vi "contatore_pulsew.vi"() -> ()   [LabVIEW 2014]
doc: "Contatore di pulse width\nFN & ADL febb 2012"
uses:
  <vilib>/DAQmx/read.llb/DAQmx Read (Counter 1D DBL 1Chan NSamp).vi
  <vilib>/Analysis/baseanly.llb/Mean (DBL).vi
  <vilib>/DAQmx/create/channels.llb/DAQmx Create Channel (CI-Pulse Width).vi
  <vilib>/DAQmx/miscellaneous.llb/DAQmx Fill In Error Info.vi
  <vilib>/Analysis/NI_AALBase.lvlib
panel:
  out "Istogramma":T1(graph)
  out "Media":dbl format="%.3e"
  in  "Azzera la figura":bool
  in  "Starting edge":i32(ring)=10280 items=["Rising"=10280, "Falling"=10171]
  in  "Numero campioni":i32=100
  out "Waveform Chart":dbl[](graph)=[857.7892626229052, 855.230805413611, 853.9527337161888, 856.0361247244633, 857.513425444567, 856.6961512925403, 855.9720097152823, 853.3515381661476, 854.4269998931967, 855.4685829162925, 858.4059401691061, 858.2401785139573, 855.2125203112975, 855.3771143853047, 855.9536929052139, 857.0540908263073, 859.4941876705559, 857.7340809915407, 855.5875212560026, 853.5245228264465, 855.8071866408499, 857.311257568451, 856.5402199167015, 856.0727661851258, 853.7704638108045, 853.4789937482665, 855.2125203112975, 858.1020926964785, 858.2493858152833, 855.8987471782089, 855.1302470257501, 856.0727661851258, 856.3018464008563, 859.2633964533904, 858.0284650943296, 856.1643835616438, 853.752241099633, 855.3771143853047, 857.5869646781368, 856.7144998929108, 856.3018464008563, 854.3631256874954, 853.4061573254252, 855.0205739325602, 857.9180473785243, 858.5164835164836, 855.9079043094964, 855.1211065267119, 855.743105919603, 856.384345294168, 859.4757198109153, 857.9548501260122, 856.3293442658046, 853.5336292249916, 854.5912917147374, 857.2010243552241, 856.9163863835986, 855.9170616367275, 854.5730339479139, 853.0239699735562, 854.4452514205153, 857.0908194859599, 857.9732526838477, 856.0269648493928, 854.8926575406877, 855.459435182908, 855.8895902428587, 858.9866105462081, 857.568578687277, 856.1368962897168, 853.4607834769993, 854.3996240641654, 856.8429621061201, 856.8888508049399, 856.2376915831835, 855.2399482579832, 853.0967411704487, 854.417874421933, 857.1275512937269, 858.5717658674795, 856.5402199167015, 854.7008547008546, 855.6058223976214, 856.3660108330301, 858.866725355893, 858.157321690999, 856.8337849561408, 853.752241099633, 854.1442008947162, 856.9990037386582, 856.9163863835986, 856.1918725986494, 855.3222426549204, 852.5512596444862, 854.5182653279215, 856.742024267218, 858.3322604180079, 856.8429621061201, 854.837847945718, 855.4045528907328]
  out "Durata":dbl[](array[numeric])=[857.7892626229052, 855.230805413611, 853.9527337161888, 856.0361247244633, 857.513425444567, 856.6961512925403, 855.9720097152823, 853.3515381661476, 854.4269998931967, 855.4685829162925, 858.4059401691061, 858.2401785139573, 855.2125203112975, 855.3771143853047, 855.9536929052139, 857.0540908263073, 859.4941876705559, 857.7340809915407, 855.5875212560026, 853.5245228264465, 855.8071866408499, 857.311257568451, 856.5402199167015, 856.0727661851258, 853.7704638108045, 853.4789937482665, 855.2125203112975, 858.1020926964785, 858.2493858152833, 855.8987471782089, 855.1302470257501, 856.0727661851258, 856.3018464008563, 859.2633964533904, 858.0284650943296, 856.1643835616438, 853.752241099633, 855.3771143853047, 857.5869646781368, 856.7144998929108, 856.3018464008563, 854.3631256874954, 853.4061573254252, 855.0205739325602, 857.9180473785243, 858.5164835164836, 855.9079043094964, 855.1211065267119, 855.743105919603, 856.384345294168, 859.4757198109153, 857.9548501260122, 856.3293442658046, 853.5336292249916, 854.5912917147374, 857.2010243552241, 856.9163863835986, 855.9170616367275, 854.5730339479139, 853.0239699735562, 854.4452514205153, 857.0908194859599, 857.9732526838477, 856.0269648493928, 854.8926575406877, 855.459435182908, 855.8895902428587, 858.9866105462081, 857.568578687277, 856.1368962897168, 853.4607834769993, 854.3996240641654, 856.8429621061201, 856.8888508049399, 856.2376915831835, 855.2399482579832, 853.0967411704487, 854.417874421933, 857.1275512937269, 858.5717658674795, 856.5402199167015, 854.7008547008546, 855.6058223976214, 856.3660108330301, 858.866725355893, 858.157321690999, 856.8337849561408, 853.752241099633, 854.1442008947162, 856.9990037386582, 856.9163863835986, 856.1918725986494, 855.3222426549204, 852.5512596444862, 854.5182653279215, 856.742024267218, 858.3322604180079, 856.8429621061201, 854.837847945718, 855.4045528907328] format="%.3e"
  # "Connettere il segnale logico \nda misurare al CB3  (Contatore 0)\ne la massa al CB12 (oppure CB13...)\nScegliere se azzerare o no la figura,\nscegliere il tipo di fronte di trigger,\npoi premere RUN."
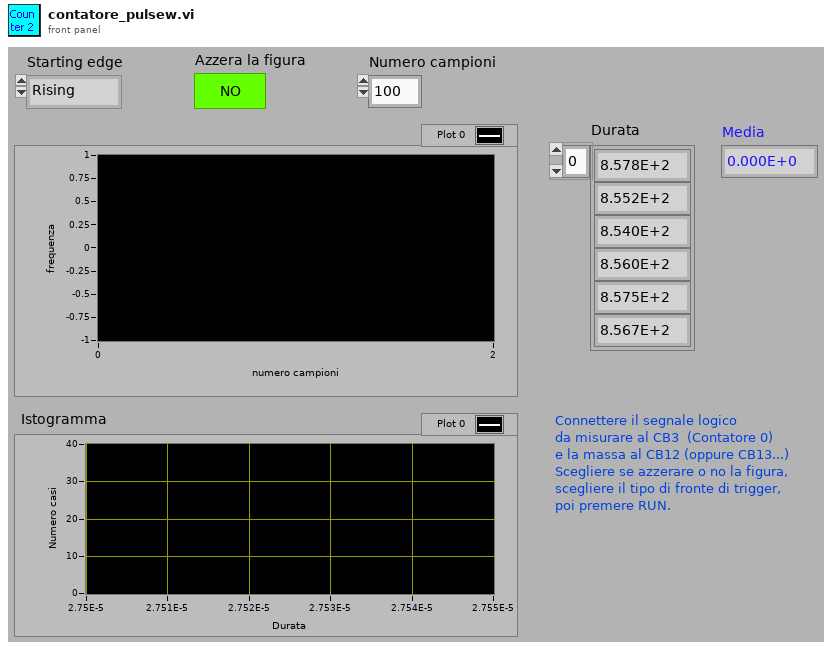
[diagram p1: front panel]
types:
  T1 = cluster{"X Values":dbl[], "Histogram: h(x)":i32[]}
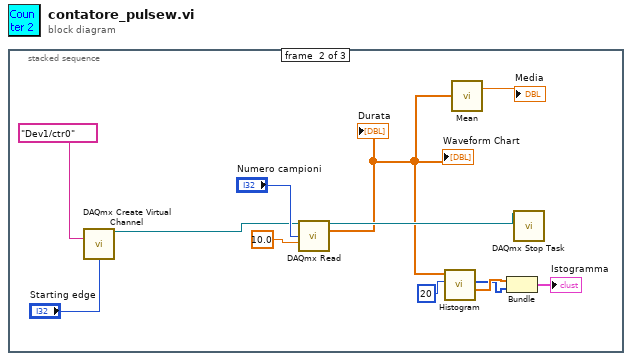
[diagram p0: block diagram]
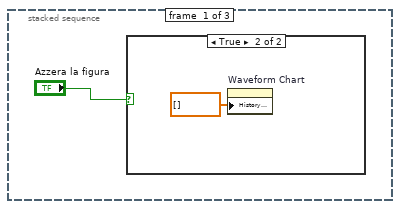
[diagram p2: hidden frame]
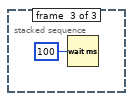
[diagram p4: hidden frame]
diagram:
  n1 = stacked-sequence {
    frame #0 {
      n2 = case shown="True" "Azzera la figura" {
        frame False {
        }
        frame True {
          n3 = property on="Waveform Chart" class="WFChart (strict)"("History Data"=dbl[] []) -> ()  [unwired: 2 in, 2 out]
        }
      }
    }
    frame #1 {
      n4 = call-poly <vilib>:"DAQmx Create Virtual Channel.vi"("counter"=tag "Dev1/ctr0" ("counter input"), "starting edge"="Starting edge") -> ("task out"=w10:refnum<k21>)  [unwired: 12 in, 1 out]
      n5 = call-poly <vilib>:"DAQmx Read.vi"("task/channels in"=w10, "number of samples per channel"="Numero campioni", "timeout"=10.0) -> ("task out"=w13:refnum<k21>, "data"=w7:dbl[])  [unwired: 10 in, 1 out]
      "Durata" <- w7
      "Waveform Chart" <- w7
      n6 = call <vilib>:"Histogram.vi"("intervals"=20, "X"=w7) -> ("X Values"=w6:dbl[], "Histogram: h(x)"=w5:i32[])  [unwired: 6 in, 2 out]
      n7 = call-poly <vilib>:"Mean.vi"("X"=w7) -> ("mean"=→"Media":dbl)  [unwired: 1 out]
      n8 = Bundle("X Values"=w6, "Histogram: h(x)"=w5) -> (→"Istogramma":T1)  [unwired: 1 in]
      n9 = call <vilib>:"DAQmx Stop Task.vi"("task/channels in"=w13) -> ()  [unwired: 13 in, 2 out]
    }
    frame #2 {
      n10 = Wait (ms)(milliseconds to wait=u32 100) -> ()  [unwired: 1 out]
    }
  }
